vi "Is Initialized.vi"(8 "Error In":errorcluster, 11 "reference in":refnum<class "Communicator.lvclass">) -> (0 "Error Out":errorcluster, 2 "Is Initialized?":bool, 3 "reference out":refnum<class "Communicator.lvclass">)   [LabVIEW 2024, in "Communicator.lvclass"]
uses:
  Communicator.lvclass
  Communicator.lvclass/Communicator.ctl
  Interfaces/IConfigure/IConfigure.lvclass
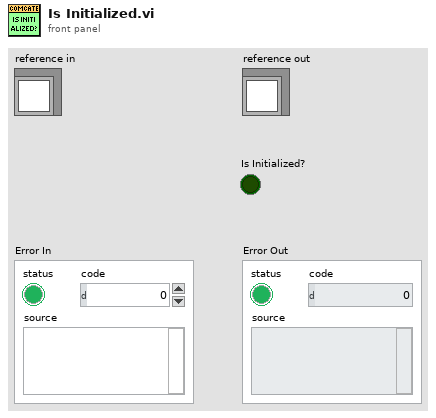
[diagram p1: front panel]
types:
  T1 = typedef "Communicator.lvclass/ObjectAttributes.ctl" = cluster{"IConfigure":refnum<class "IConfigure.lvclass">, "Worker Enqueuer":refnum<class "Message Enqueuer.lvclass">, "Start Counter":i32, "Msg Sent":refnum<user-event>}
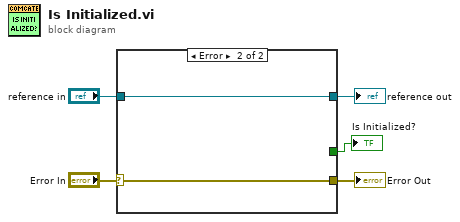
[diagram p0: block diagram]
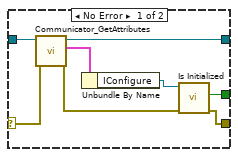
[diagram p2: hidden frame]
diagram:
  n1 = case shown="Error" "Error In" {
    selector: "Error In" -> [w13 w15]
    tunnel: [w7 w15] -> w4
    tunnel: [w10 w14] -> w2
    tunnel: "reference in" -> [w11 w14]
    tunnel: [w6 _] -> w1
    frame No Error {
      n2 = call "Communicator_GetAttributes.vi"("Error In"=w13, "Communicator in"=w11) -> ("Error Out"=w8:errorcluster, "Data"=w12:T1, "Communicator out"=w10:refnum<class "Communicator.lvclass">)  [unwired: 6 in, 1 out]
      n3 = Unbundle By Name(w12) -> ("IConfigure"=w9:refnum<class "IConfigure.lvclass">)
      n4 = call-dynamic "Is Initialized.vi"("error in"=w8, "IInitialize in"=w9) -> ("error out"=w7:errorcluster, "Is Initialized?"=w6:bool)  [unwired: 7 in, 1 out]
    }
    frame Error {
    }
  }
  "Error Out" <- w4
  "reference out" <- w2
  "Is Initialized?" <- w1
